vi "readInFile.vi"(8 "error in (no error)":errorcluster, 10 "Path":path=path "C:/Users/Administrator/Desktop/Crete/Data/2014/1411/141126/Scripts/Instrument Scripts/Dio64.csv", 11 "FileReader in":refnum<class "FileReader.lvclass">) -> (0 "error out":errorcluster, 3 "FileReader out":refnum<class "FileReader.lvclass">)   [LabVIEW 2011, in "Tools.lvlib" / "Filing.lvlib" / "FileReader.lvclass"]
uses:
  FileReader.lvclass
  Ao8/Ao8FileReader.lvclass
  Dio64/Dio64FileReader.lvclass
  K2602/K2602FileReader.lvclass
  DDS/DDSFileReader.lvclass
  k3390/K3390FileReader.lvclass
  FileReader.lvclass/FileReader.ctl
panel:
  out "config":string
  out "data":string
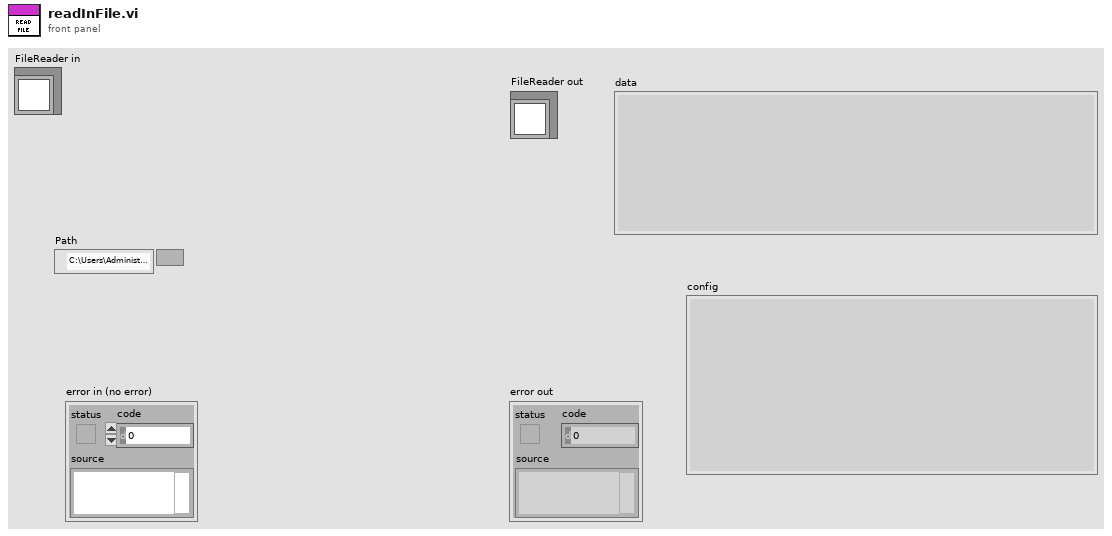
[diagram p1: front panel]
types:
  T1 = cluster{"aoChannels":refnum<class "AnalogOutput.lvclass">[], "doChannels":refnum<class "DigitalOutput.lvclass">[], "rfChannels":refnum<class "DDSOutput.lvclass">[]}
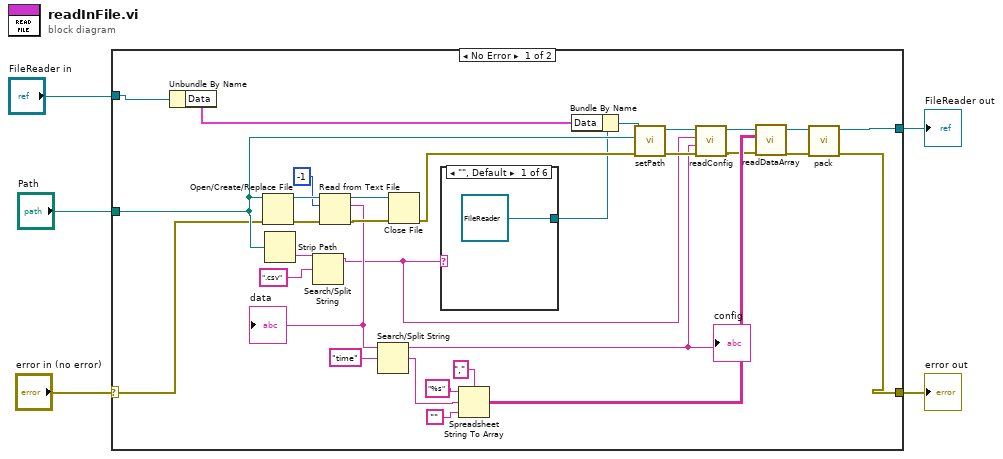
[diagram p0: block diagram]
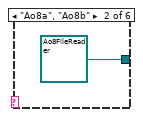
[diagram p2: hidden frame]
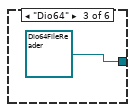
[diagram p3: hidden frame]
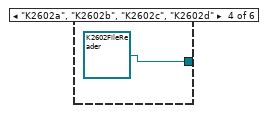
[diagram p4: hidden frame]
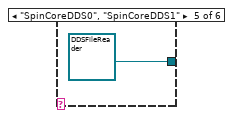
[diagram p5: hidden frame]
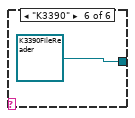
[diagram p6: hidden frame]
diagram:
  n1 = case shown="No Error" "error in (no error)" {
    selector: "error in (no error)" -> [w22 w43]
    tunnel: [w6 w43] -> w4
    tunnel: [w8 _] -> w3
    tunnel: "Path" -> [w23 _]
    tunnel: "FileReader in" -> [w13 _]
    frame No Error {
      n2 = Unbundle By Name(w13) -> ("Data"=w10:T1)
      n3 = Open/Create/Replace File(file path (use dialog)=w23, error in=w22) -> (refnum out=w36:refnum<file>, error out=w32:errorcluster)  [unwired: 4 in, 1 out]
      n4 = Strip Path(path=w23) -> (name=w26:string)  [unwired: 1 out]
      n5 = Search/Split String(string=w26, search string/char (-)=".csv") -> (substring before match=w14:string)  [unwired: 1 in, 2 out]
      n6 = Read from Text File(file (use dialog)=w36, count=-1, error in=w32) -> (refnum out=w35:refnum<file>, text=w24:string, error out=w33:errorcluster)  [unwired: 1 in, 1 out]
      "data" <- w24
      n7 = Search/Split String(string=w24, search string/char (-)="time") -> (substring before match=w15:string, match + rest of string=w28:string)  [unwired: 1 in, 1 out]
      "config" <- w15
      n8 = Close File(refnum=w35, error in=w33) -> (error out=w21:errorcluster)  [unwired: 1 out]
      n9 = case shown="\"\", Default" w14 {
        tunnel: [refnum<class "FileReader.lvclass"> refnum ("Tools.lvlib:Filing.lvlib:FileReader.lvclass") refnum<class "Ao8FileReader.lvclass"> refnum ("Tools.lvlib:Filing.lvlib:Ao8FileReader.lvclass") refnum<class "Dio64FileReader.lvclass"> refnum ("Tools.lvlib:Filing.lvlib:Dio64FileReader.lvclass") refnum<class "K2602FileReader.lvclass"> refnum ("Tools.lvlib:Filing.lvlib:K2602FileReader.lvclass") refnum<class "DDSFileReader.lvclass"> refnum ("Tools.lvlib:Filing.lvlib:SpinCoreDDSFileReader.lvclass") refnum<class "K3390FileReader.lvclass"> refnum ("Tools.lvlib:Filing.lvlib:K3390FileReader.lvclass")] -> w12
        frame "", Default {
        }
        frame "Ao8a", "Ao8b" {
        }
        frame "Dio64" {
        }
        frame "K2602a", "K2602b", "K2602c", "K2602d" {
        }
        frame "SpinCoreDDS0", "SpinCoreDDS1" {
        }
        frame "K3390" {
        }
      }
      n10 = Spreadsheet String To Array(delimiter (Tab)=",", format string="%s", spreadsheet string=w28, array type (2D Dbl)="") -> (array=w17:string[][])
      n11 = Bundle By Name(cluster=w12, "Data"=w10) -> (w11:refnum<class "FileReader.lvclass">)
      n12 = call "setPath.vi"("error in (no error)"=w21, "Path"=w23, "FileReader in"=w11) -> ("error out"=w19:errorcluster, "FileReader out"=w20:refnum<class "FileReader.lvclass">)  [unwired: 7 in]
      n13 = call-dynamic "readConfig.vi"("error in (no error)"=w19, "config"=w15, "deviceName"=w14, "FileReader in"=w20) -> ("error out"=w16:errorcluster, "FileReader out"=w18:refnum<class "FileReader.lvclass">)  [unwired: 6 in]
      n14 = call-dynamic "readDataArray.vi"("error in (no error)"=w16, "array"=w17, "FileReader in"=w18) -> ("error out"=w7:errorcluster, "FileReader out"=w9:refnum<class "FileReader.lvclass">)  [unwired: 7 in]
      n15 = call-dynamic "pack.vi"("error in (no error)"=w7, "FileReader in"=w9) -> ("error out"=w6:errorcluster, "FileReader out"=w8:refnum<class "FileReader.lvclass">)  [unwired: 8 in]
    }
    frame Error {
    }
  }
  "error out" <- w4
  "FileReader out" <- w3
